vi "Test MQTT-2.3.1-1.vi"(8 "error in (no error)":errorcluster) -> (0 "error out":errorcluster)   [LabVIEW 2013]
uses:
  source/Control Packets/SUBSCRIBE/Topic Subscription -- cluster.ctl
  source/Control Packets/ControlPacket/QualityOfService -- enum.ctl
  source/Control Packets/ControlPacket/ControlPacket.lvclass/ControlPacket.ctl
  <vilib>/addons/_JKI Toolkits/Caraya/classes/Test/Test.lvclass
  <vilib>/addons/_JKI Toolkits/Caraya/classes/Assert/Assert.lvclass
  source/Control Packets/PUBLISH/PUBLISH.lvclass
  source/Control Packets/SUBSCRIBE/SUBSCRIBE.lvclass
  source/Control Packets/UNSUBSCRIBE/UNSUBSCRIBE.lvclass
  source/Control Packets/ControlPacket/ControlPacket.lvclass
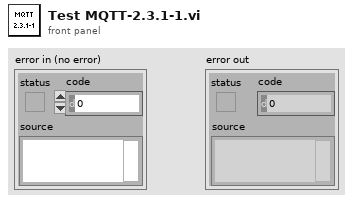
[diagram p1: front panel]
types:
  T1 = typedef "ControlPacket.lvclass/QualityOfService -- enum.ctl" = enum16{"0 (At Most Once)", "1 (At Least Once)", "2 (Exactly Once)"}
  T2 = typedef "SUBSCRIBE.lvclass/Topic Subscription -- cluster.ctl" = cluster{"Topic Filter":string, "QoS":T1}
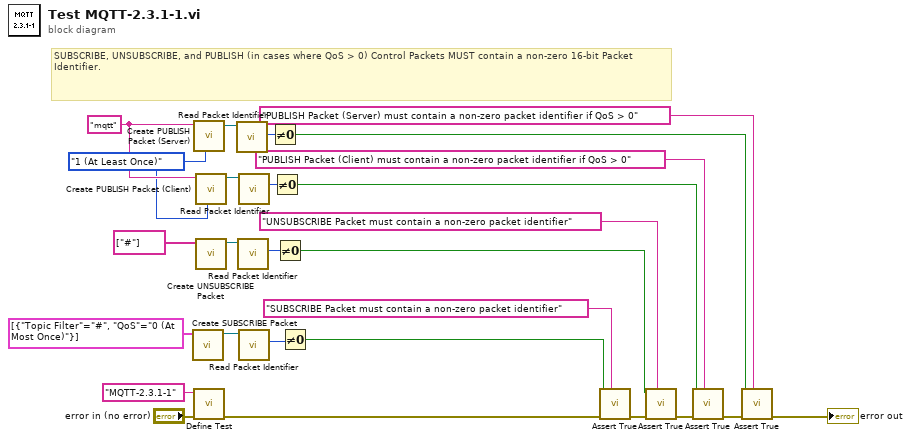
[diagram p0: block diagram]
diagram:
  w1 = QualityOfService_--_enum."1 (At Least Once)" ("QoS")
  w6 = "mqtt" ("Topic Name")
  # "SUBSCRIBE, UNSUBSCRIBE, and PUBLISH (in cases where QoS > 0) Control Packets MUST contain a non-zero 16-bit Packet Identifier."
  n1 = call "Create SUBSCRIBE Packet.vi"("Topic Subscriptions"=T2[] [{"Topic Filter"="#", "QoS"=enum."0 (At Most Once)"}]) -> ("SUBSCRIBE out"=w23:refnum<class "SUBSCRIBE.lvclass">)  [unwired: 9 in, 1 out]
  n2 = call "Create PUBLISH Packet (Server).vi"("QoS"=w1, "Topic Name"=w6) -> ("PUBLISH"=w13:refnum<class "PUBLISH.lvclass">)  [unwired: 7 in, 2 out]
  n3 = call <vilib>:"Define Test.vi"("error in (no error)"="error in (no error)", "Label (VI Title)"="MQTT-2.3.1-1") -> ("error out"=w24:errorcluster)  [unwired: 9 in]
  n4 = call "Create PUBLISH Packet (Client).vi"("QoS"=w1, "Topic Name"=w6) -> ("PUBLISH"=w14:refnum<class "PUBLISH.lvclass">)  [unwired: 7 in, 2 out]
  n5 = call "Create UNSUBSCRIBE Packet.vi"("Topic Subscriptions"=string[] ["#"]) -> ("UNSUBSCRIBE out"=w15:refnum<class "UNSUBSCRIBE.lvclass">)  [unwired: 9 in, 1 out]
  n6 = call "Read Packet Identifier.vi"("ControlPacket in"=w13) -> ("Packet Identifier"=w10:u16)  [unwired: 9 in, 1 out]
  n7 = call "Read Packet Identifier.vi"("ControlPacket in"=w15) -> ("Packet Identifier"=w12:u16)  [unwired: 9 in, 1 out]
  n8 = call "Read Packet Identifier.vi"("ControlPacket in"=w14) -> ("Packet Identifier"=w11:u16)  [unwired: 9 in, 1 out]
  n9 = call "Read Packet Identifier.vi"("ControlPacket in"=w23) -> ("Packet Identifier"=w22:u16)  [unwired: 9 in, 1 out]
  n10 = Not Equal To 0?(x=w10) -> (x != 0?=w7:bool)
  n11 = Not Equal To 0?(x=w11) -> (x != 0?=w8:bool)
  n12 = Not Equal To 0?(x=w12) -> (x != 0?=w9:bool)
  n13 = Not Equal To 0?(x=w22) -> (x != 0?=w21:bool)
  n14 = call <vilib>:"Assert True.vi"("Label"="SUBSCRIBE Packet must contain a non-zero packet identifier", "error in (no error)"=w24, "True?"=w21) -> ("error out"=w19:errorcluster)  [unwired: 8 in]
  n15 = call <vilib>:"Assert True.vi"("Label"="UNSUBSCRIBE Packet must contain a non-zero packet identifier", "error in (no error)"=w19, "True?"=w9) -> ("error out"=w18:errorcluster)  [unwired: 8 in]
  n16 = call <vilib>:"Assert True.vi"("Label"="PUBLISH Packet (Client) must contain a non-zero packet identifier if QoS > 0", "error in (no error)"=w18, "True?"=w8) -> ("error out"=w17:errorcluster)  [unwired: 8 in]
  n17 = call <vilib>:"Assert True.vi"("Label"="PUBLISH Packet (Server) must contain a non-zero packet identifier if QoS > 0", "error in (no error)"=w17, "True?"=w7) -> ("error out"=→"error out":errorcluster)  [unwired: 8 in]
